vi "Update Bind Methods.vi"(7 "RPC Method Parameters":T1[](array[typedef]), 8 "error in (no error)":errorcluster, 11 "Server class in":refnum<vi>) -> (0 "error out":errorcluster, 3 "Server class out":refnum<vi>)   [LabVIEW 2019, in "gRPC Scripting Tools.lvlib"]
uses:
  gRPC Scripting Tools.lvlib
  TypeDefs/RPC Method Parameters.ctl
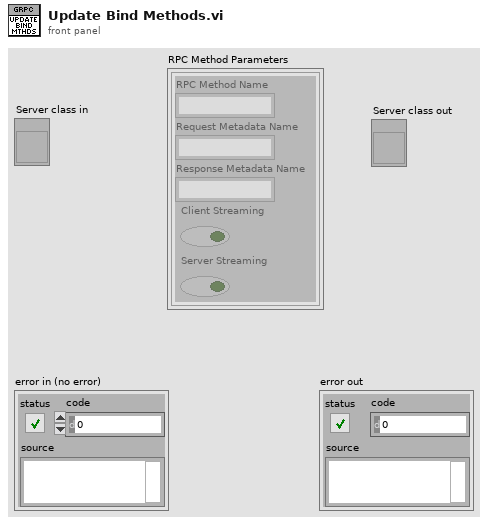
[diagram p1: front panel]
types:
  T1 = typedef "gRPC Scripting Tools.lvlib/RPC Method Parameters.ctl" = cluster{"RPC Method Name":string, "Request Metadata Name":string, "Response Metadata Name":string, "Client Streaming":bool, "Server Streaming":bool}
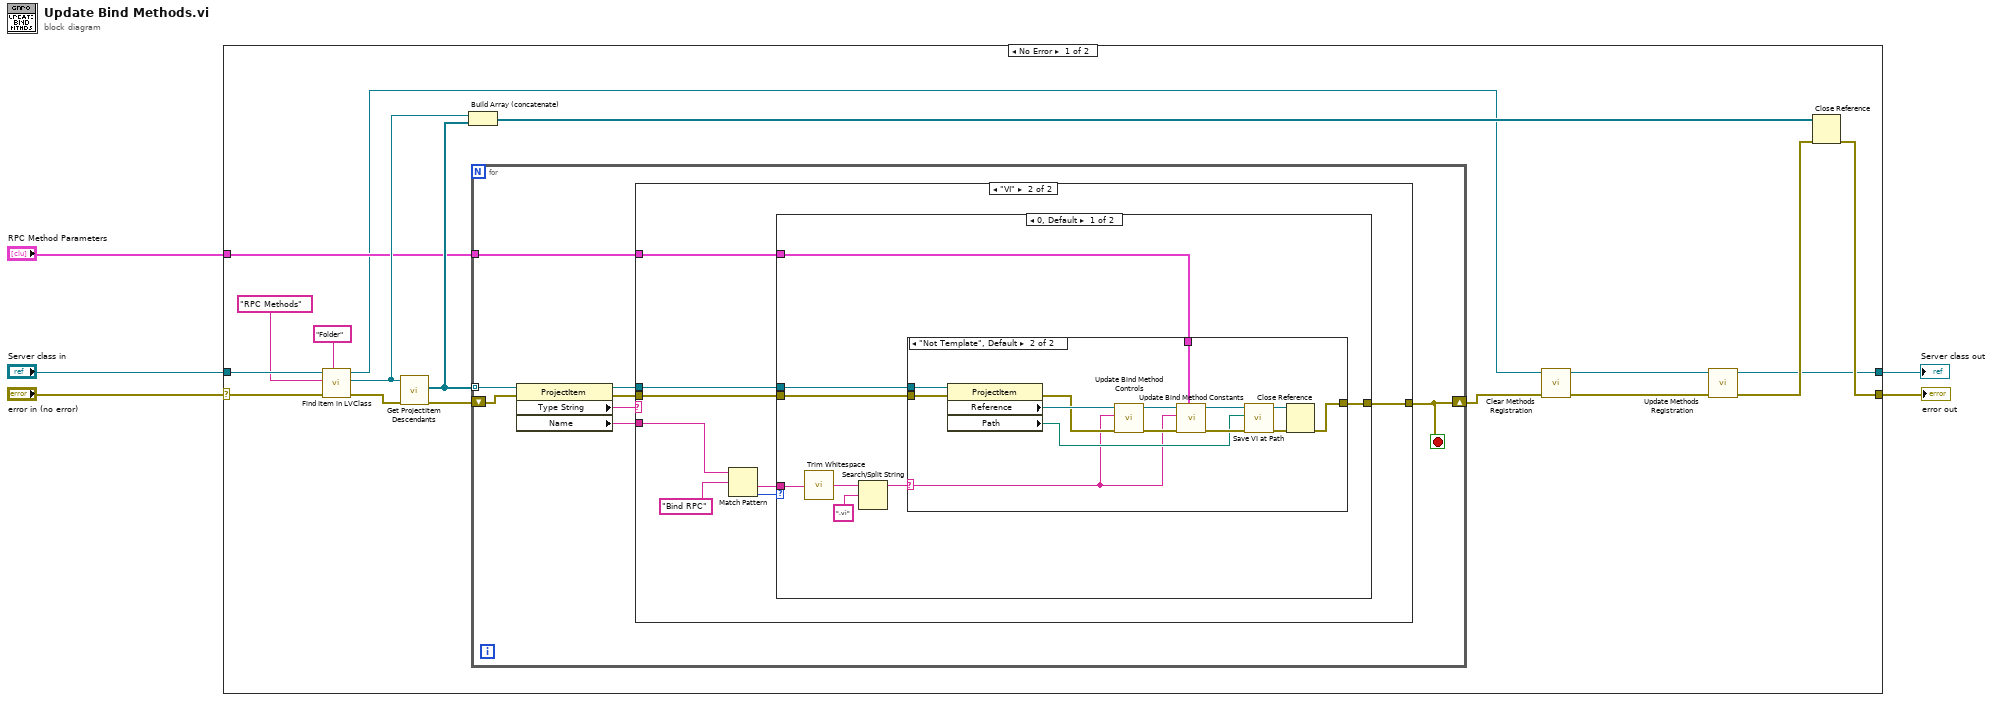
[diagram p0: block diagram]
diagram:
  n1 = case shown="No Error" "error in (no error)" {
    selector: "error in (no error)" -> [w13 w65]
    tunnel: [w7 w65] -> w5
    tunnel: "Server class in" -> [w17 w64]
    tunnel: "RPC Method Parameters" -> [w14 _]
    tunnel: [w6 w64] -> w1
    frame No Error {
      n2 = call "Find Item in LVClass.vi"("Item Type"="Folder", "error in (no error)"=w13, "Item Name"="RPC Methods", "Class Item in"=w17) -> ("error out"=w18:errorcluster, "Project Item (Class Item)"=w19:refnum<vi>, "Class Item out"=w9:refnum<vi>)  [unwired: 4 in, 1 out]
      n3 = call "Get ProjectItem Descendants.vi"("error in (no error)"=w18, "ProjectItem in"=w19) -> ("error out"=w22:errorcluster, "All Descendents"=w20:refnum<vi>[])  [unwired: 7 in, 1 out]
      n4 = Build Array (concatenate)(w19, w20) -> (w21:refnum<vi>[])
      n5 = for {
        tunnel: w20 -> [w30] mode=indexing
        shift-right: [w24] -> w10
        shift-left: w22 -> [w27]
        tunnel: w14 -> [w23]
        stop <- w24 stop-if-true
        n6 = property class="ProjectItem"(reference=w30, error in=w27) -> (reference out=w28:refnum<vi>, error out=w26:errorcluster, "Type String"=w29:string, "Name"=w25:string)
        n7 = case shown="\"VI\"" w29 {
          tunnel: w28 -> [_ w37]
          tunnel: w26 -> [w31 w35]
          tunnel: w25 -> [_ w33]
          tunnel: [w31 w36] -> w24
          tunnel: w23 -> [_ w32]
          frame "None", Default {
          }
          frame "VI" {
            n8 = Match Pattern(string=w33, regular expression="Bind RPC") -> (after substring=w34:string, offset past match=w38:i32)  [unwired: 1 in, 2 out]
            n9 = case shown="0, Default" w38 {
              tunnel: w37 -> [w47 _]
              tunnel: [w44 w63] -> w36
              tunnel: w35 -> [w46 w63]
              tunnel: w34 -> [w43 _]
              tunnel: w32 -> [w45 _]
              frame 0, Default {
                n10 = call <vilib>:"Trim Whitespace.vi"("string"=w43) -> ("trimmed string"=w42:string)  [unwired: 1 in]
                n11 = Search/Split String(string=w42, search string/char (-)=".vi" ("regular expression")) -> (substring before match=w40:string)  [unwired: 1 in, 2 out]
                n12 = case shown="\"Not Template\", Default" w40 {
                  selector: w40 -> [_ w49]
                  tunnel: w47 -> [_ w62]
                  tunnel: w46 -> [w48 w61]
                  tunnel: w45 -> [_ w56]
                  tunnel: [w48 w55] -> w44
                  frame "Template" {
                  }
                  frame "Not Template", Default {
                    n13 = property class="ProjectItem"(reference=w62, error in=w61) -> (error out=w59:errorcluster, "Reference"=w60:refnum<vi>, "Path"=w50:path)  [unwired: 1 out]
                    n14 = call "Update Bind Method Controls.vi"("error in (no error)"=w59, "Method Name"=w49, "VI in"=w60) -> ("error out"=w58:errorcluster, "VI out"=w57:refnum<vi>)  [unwired: 7 in]
                    n15 = call "Update Bind Method Constants.vi"("RPC Method Parameters"=w56, "error in (no error)"=w58, "RPC Method Name"=w49, "VI in"=w57) -> ("error out"=w54:errorcluster, "VI out"=w51:refnum<vi>)  [unwired: 6 in]
                    n16 = call "Save VI at Path.vi"("error in (no error)"=w54, "Path"=w50, "VI in"=w51) -> ("error out"=w53:errorcluster, "VI out"=w52:refnum<vi>)  [unwired: 6 in, 1 out]
                    n17 = Close Reference(reference=w52, error in (no error)=w53) -> (error out=w55:errorcluster)
                  }
                }
              }
              frame -1 {
              }
            }
          }
        }
      }
      n18 = call "Clear Methods Registration.vi"("error in (no error)"=w10, "Server class in"=w9) -> ("error out"=w12:errorcluster, "Server class out"=w11:refnum<vi>)  [unwired: 8 in]
      n19 = call "Update Methods Registration.vi"("error in (no error)"=w12, "Server class in"=w11) -> ("error out"=w8:errorcluster, "Server class out"=w6:refnum<vi>)  [unwired: 8 in]
      n20 = Close Reference(reference=w21, error in (no error)=w8) -> (error out=w7:errorcluster)
    }
    frame Error {
    }
  }
  "error out" <- w5
  "Server class out" <- w1
